vi "add_error_in_out.vi"() -> ()   [LabVIEW 2020]
uses:
  <vilib>/Utility/miscctls.llb/LVPointTypeDef.ctl
panel:
  out "error out":errorcluster
  out "path":path
  out "text":string
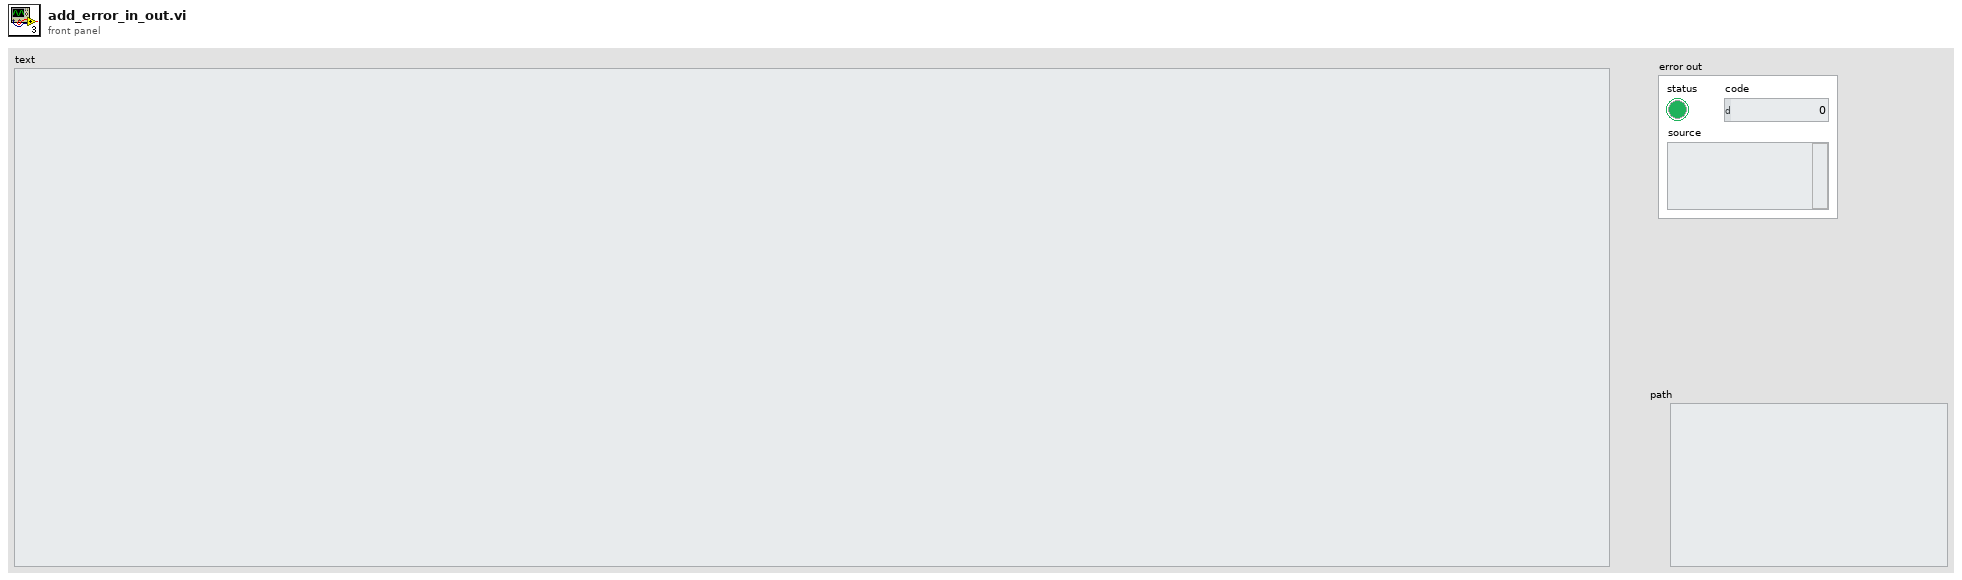
[diagram p1: front panel]
types:
  T1 = enum16{"open", "replace", "create", "open or create", "replace or create", "replace or create with confirmation"}
  T2 = typedef "LVPointTypeDef.ctl" = cluster{"Horizontal":i16, "Vertical":i16}
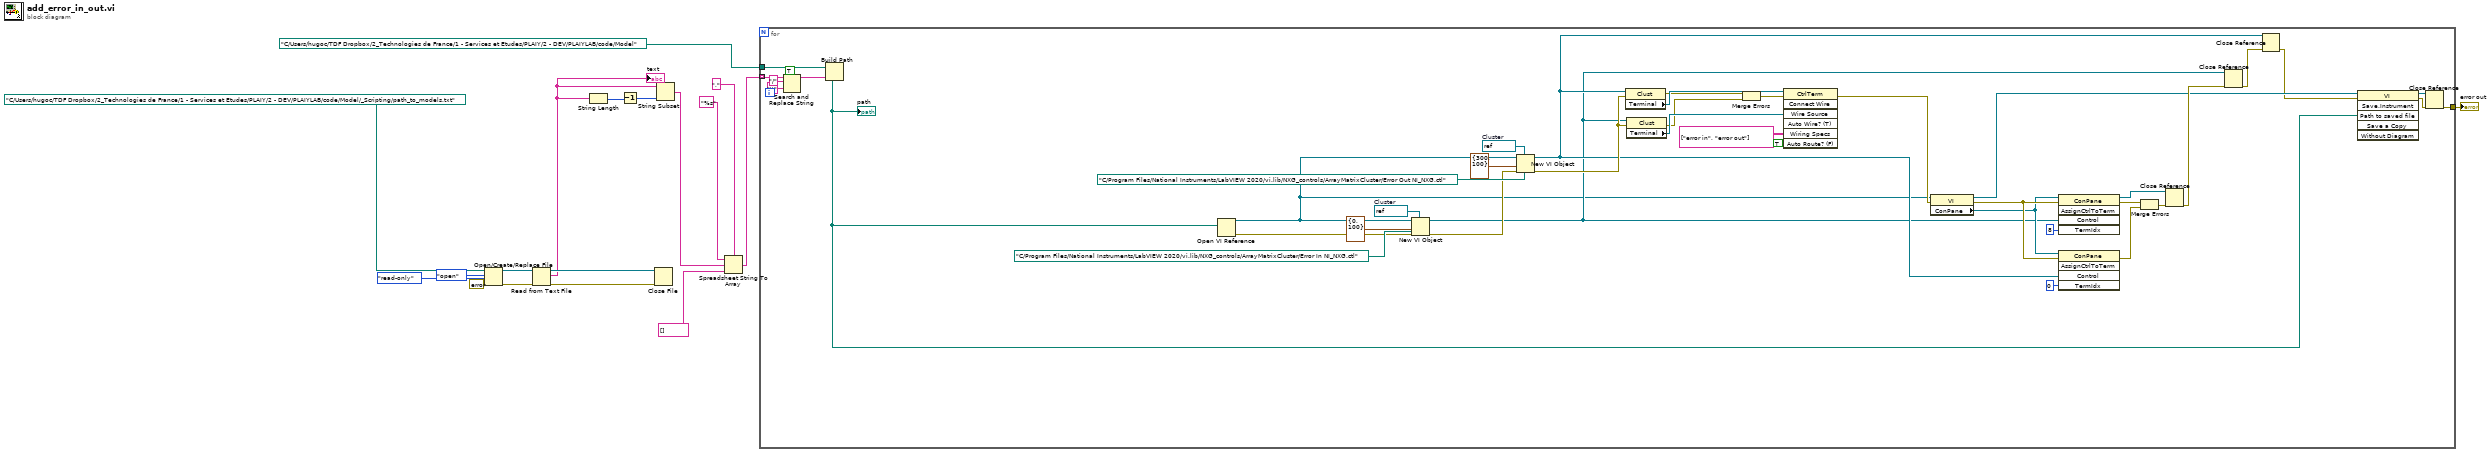
[diagram p0: block diagram]
diagram:
  n1 = Open/Create/Replace File(file path (use dialog)=path "C:/Users/hugoc/TDF Dropbox/2_Technologies de France/1 - Services et Etudes/PLAIY/2 - DEV/PLAIYLAB/code/Model/_Scripting/path_to_models.txt", error in=errorcluster {"status"=FALSE, "code"=0, "source"=""}, operation (0:open)=T1."open", access (0:read/write)=enum16{"read/write", "read-only", "write-only"}."read-only") -> (refnum out=w14:refnum<file>, error out=w13:errorcluster)  [unwired: 2 in, 1 out]
  n2 = Read from Text File(file (use dialog)=w14, error in=w13) -> (refnum out=w12:refnum<file>, text=w4:string, error out=w11:errorcluster)  [unwired: 2 in, 1 out]
  "text" <- w4
  n3 = String Length(string=w4) -> (length=w3:i32)
  n4 = Decrement(x=w3) -> (x-1=w2:i32)
  n5 = Close File(refnum=w12, error in=w11) -> ()  [unwired: 2 out]
  n6 = String Subset(string=w4, length (rest)=w2) -> (substring=w5:string)  [unwired: 1 in]
  n7 = Spreadsheet String To Array(delimiter (Tab)=",", format string="%s", spreadsheet string=w5, array type (2D Dbl)=string[] []) -> (array=w7:string[])
  n8 = for {
    tunnel: w7 -> [w58] mode=indexing
    tunnel: path "C:/Users/hugoc/TDF Dropbox/2_Technologies de France/1 - Services et Etudes/PLAIY/2 - DEV/PLAIYLAB/code/Model" -> [w60]
    tunnel: [w19] -> w1
    w48 = refnum<vi> refnum  # Cluster
    w52 = refnum<vi> refnum  # Cluster
    n9 = Search and Replace String(replace all?=TRUE ("replace all? (F)"), input string=w58, search string="/", replace string="\\" ("replace string (\"\")")) -> (result string=w55:string)  [unwired: 4 in, 3 out]
    n10 = Build Path(base path=w60, name or relative path=w55) -> (appended path=w22:path)
    "path" <- w22
    n11 = Open VI Reference(vi path=w22) -> (vi reference=w24:refnum<vi>, error out=w23:errorcluster)  [unwired: 5 in]
    n12 = New VI Object(vi object class=w52, owner refnum=w24, position/next to=T2 {"Horizontal"=0, "Vertical"=100} ("location"), 6:path "C:/Program Files/National Instruments/LabVIEW 2020/vi.lib/NXG_controls/ArrayMatrixCluster/Error In NI_NXG.ctl" ("path"), 8:w23) -> (object refnum=w26:refnum<vi>, 0:w44:errorcluster)  [unwired: 3 in]
    n13 = New VI Object(vi object class=w48, owner refnum=w24, position/next to=T2 {"Horizontal"=300, "Vertical"=100} ("location"), 6:path "C:/Program Files/National Instruments/LabVIEW 2020/vi.lib/NXG_controls/ArrayMatrixCluster/Error Out NI_NXG.ctl" ("path"), 8:w44) -> (object refnum=w27:refnum<vi>, 0:w36:errorcluster)  [unwired: 3 in]
    n14 = property class="Clust"(reference=w27, error in=w36) -> (error out=w34:errorcluster, "Terminal"=w39:refnum<vi>)  [unwired: 1 out]
    n15 = property class="Clust"(reference=w26, error in=w36) -> (error out=w33:errorcluster, "Terminal"=w38:refnum<vi>)  [unwired: 1 out]
    n16 = Merge Errors(w34, w33) -> (w35:errorcluster)
    n17 = invoke class="CtrlTerm" method="Connect Wire"(reference=w39, error in=w35, "Wire Source"=w38, "Wiring Specs"=string[][] [["error in", "error out"]], "Auto Route? (F)"=TRUE) -> (error out=w31:errorcluster)  [unwired: 2 in, 6 out]
    n18 = property class="VI"(reference=w24, error in=w31) -> (reference out=w21:refnum<vi>, error out=w43:errorcluster, "ConPane"=w40:refnum<vi>)
    n19 = invoke class="ConPane" method="AssignCtrlToTerm"(reference=w40, error in=w43, "Control"=w26, "TermIdx"=u32 8 ("Terminal Index")) -> (reference out=w30:refnum<vi>, error out=w42:errorcluster)  [unwired: 1 in, 3 out]
    n20 = invoke class="ConPane" method="AssignCtrlToTerm"(reference=w40, error in=w43, "Control"=w27, "TermIdx"=u32 0 ("Terminal Index")) -> (error out=w41:errorcluster)  [unwired: 1 in, 4 out]
    n21 = Merge Errors(w42, w41) -> (w29:errorcluster)
    n22 = Close Reference(reference=w30, error in (no error)=w29) -> (error out=w28:errorcluster)
    n23 = Close Reference(reference=w26, error in (no error)=w28) -> (error out=w25:errorcluster)
    n24 = Close Reference(reference=w27, error in (no error)=w25) -> (error out=w20:errorcluster)
    n25 = invoke class="VI" method="Save.Instrument"(reference=w21, error in=w20, "Path to saved file"=w22) -> (reference out=w54:refnum<vi>, error out=w53:errorcluster)  [unwired: 3 in, 4 out]
    n26 = Close Reference(reference=w54, error in (no error)=w53) -> (error out=w19:errorcluster)
  }
  "error out" <- w1
